vi "GetSerialPortList.vi"(8 "error in (no error)":errorcluster caption="错误输入（无错误）") -> (0 "error out":errorcluster caption="错误输出", 1 "pSerialPortList":T1(array[cluster]), 2 "function return":i32)   [LabVIEW 2013, in "MvCameraControl.lvlib"]
doc: "MV_LV_API int __stdcall GetStringValue( void* handle, const char* strKey, MVCC_STRINGVALUE *pStringValue);"
uses:
  MvCameraControl.lvlib
  MvCameraPatch.dll
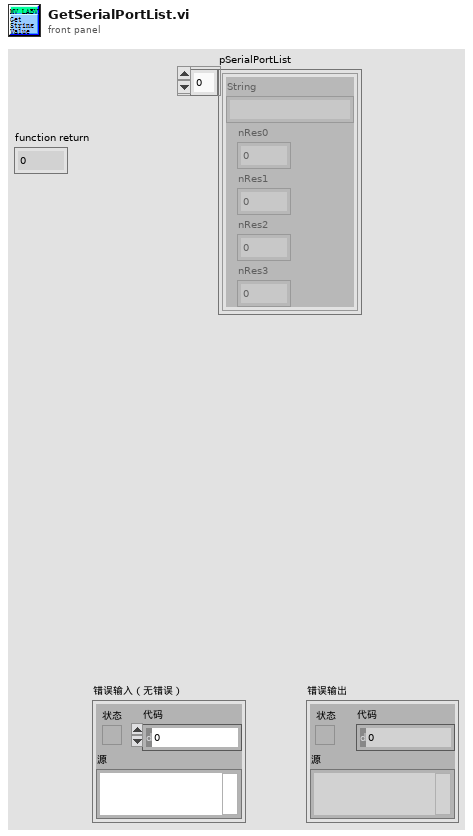
[diagram p1: front panel]
types:
  T1 = cluster{"String":string, "nRes0":u32, "nRes1":u32, "nRes2":u32, "nRes3":u32}[]
  T2 = cluster{"String":string, "nRes0":u32, "nRes1":u32, "nRes2":u32, "nRes3":u32}
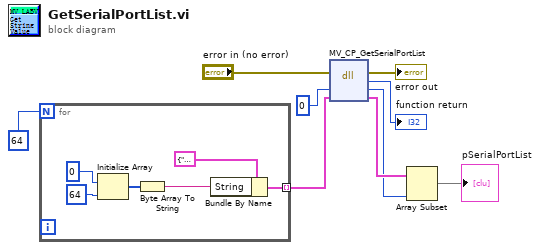
[diagram p0: block diagram]
diagram:
  n1 = for {
    N: 64 -> [_]
    tunnel: [w10] -> w4 mode=indexing
    n2 = Initialize Array(u8 0 ("element"), 64) -> (w13:u8[])
    n3 = Byte Array To String(unsigned byte array=w13) -> (string=w12:string)
    n4 = Bundle By Name(cluster=T2 {"String"="", "nRes0"=0, "nRes1"=0, "nRes2"=0, "nRes3"=0} ("CMLSerialPort"), "String"=w12) -> (w10:T2)
  }
  n5 = dll-call lib="MvCameraPatch.dll" fn="MV_CP_GetSerialPortList"(error in="error in (no error)", "nSerialPortNum"=u32 0, "pSerialPortList"=w4) -> (error out=→"error out":errorcluster, "返回类型"=→"function return":i32, "nSerialPortNum"=w2:u32, "pSerialPortList"=w3:T1)  [unwired: 2 in, 1 out]
  n6 = Array Subset(array=w3, length=w2) -> (→"pSerialPortList":T1)  [unwired: 1 in]
